vi "Main.vi"() -> ()   [LabVIEW 2019]
panel:
  in  "stop":bool
  out "Salida":dbl
  in  "Entrada":dbl(knob) scale=0.0..10.0
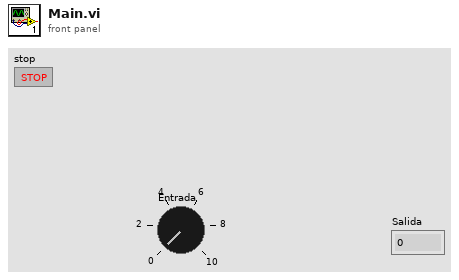
[diagram p1: front panel]
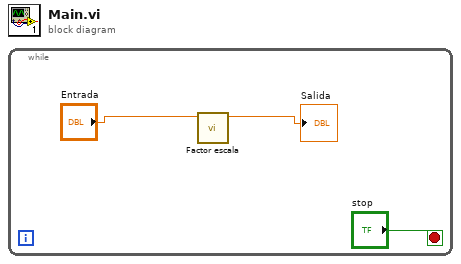
[diagram p0: block diagram]
diagram:
  n1 = while {
    stop <- "stop" stop-if-true
    n2 = call "Factor escala.vi"("Entrada"="Entrada") -> ("Numeric"=→"Salida":dbl)  [unwired: 10 in]
  }
